vi "Read Configuration.vi"(0 "VISA resource name":refnum<visa-resource-name>, 11 "error in (no error)":errorcluster) -> (1 "function":i32(ring) items=["volts DC", "volts AC", "2-wire k.ohms", "4-wire k.ohms", "mA DC", "mA AC"], 3 "range":i32(ring) items=["200mV, 200 ohms", "2V, 2 kohms", "20V, 20 kohms", "200V, 200 kohms", "1000Vdc, 700 Vac, 2 Mohms", "20 Mohms"], 4 "VISA resource name out":refnum<visa-resource-name>, 6 "offset":bool, 10 "autorange":bool, 12 "rate":i32(ring) items=["slow", "medium", "fast"], 14 "trigger mode":i32(ring) items=["internal - continuous trigger", "external - rear panel trigger with delay", "external - bus trigger with delay", "external - rear panel trigger", "external - bus trigger"], 15 "error out":errorcluster)   [LabVIEW 2017, in "Fluke 8840.lvlib"]
doc: "This VI reads the current configuration of the multimeter."
uses:
  Fluke 8840.lvlib
panel:
  out "inputs":bool
  # "on\noff"
  # "rear\nfront"
  # "on\noff"
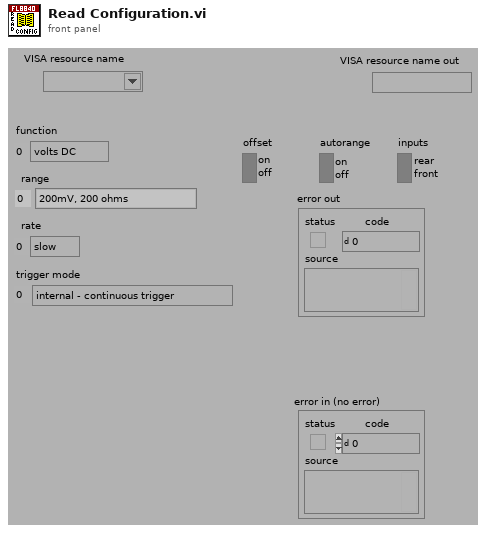
[diagram p1: front panel]
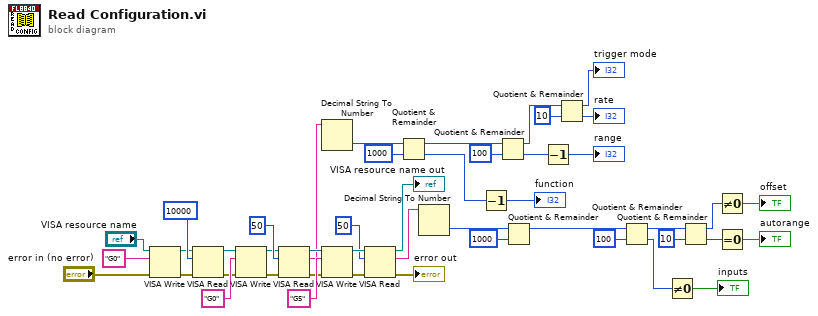
[diagram p0: block diagram]
diagram:
  n1 = VISA Write(VISA resource name="VISA resource name", write buffer="G0", error in (no error)="error in (no error)") -> (VISA resource name out=w4:refnum<visa-resource-name>, error out=w2:errorcluster)  [unwired: 1 out]
  n2 = VISA Read(VISA resource name=w4, byte count=u32 10000, error in (no error)=w2) -> (VISA resource name out=w3:refnum<visa-resource-name>, error out=w1:errorcluster)  [unwired: 2 out]
  n3 = VISA Write(VISA resource name=w3, write buffer="G0", error in (no error)=w1) -> (VISA resource name out=w13:refnum<visa-resource-name>, error out=w14:errorcluster)  [unwired: 1 out]
  n4 = VISA Read(VISA resource name=w13, byte count=u32 50, error in (no error)=w14) -> (VISA resource name out=w11:refnum<visa-resource-name>, read buffer=w10:string, error out=w12:errorcluster)  [unwired: 1 out]
  n5 = Decimal String To Number(string=w10) -> (number=w40:i32)  [unwired: 3 out]
  n6 = VISA Write(VISA resource name=w11, write buffer="G5", error in (no error)=w12) -> (VISA resource name out=w46:refnum<visa-resource-name>, error out=w45:errorcluster)  [unwired: 1 out]
  n7 = VISA Read(VISA resource name=w46, byte count=u32 50, error in (no error)=w45) -> (VISA resource name out=→"VISA resource name out":refnum<visa-resource-name>, read buffer=w9:string, error out=→"error out":errorcluster)  [unwired: 1 out]
  n8 = Quotient & Remainder(x=w40, y=1000) -> (x-y*floor(x/y)=w36:i32, floor(x/y)=w21:i32)
  n9 = Decimal String To Number(string=w9) -> (number=w27:i32)  [unwired: 3 out]
  n10 = Decrement(x=w21) -> (x-1=→"function":i32)
  n11 = Quotient & Remainder(x=w36, y=100) -> (x-y*floor(x/y)=w35:i32, floor(x/y)=w19:i32)
  n12 = Quotient & Remainder(x=w27, y=1000) -> (x-y*floor(x/y)=w29:i32)  [unwired: 1 out]
  n13 = Decrement(x=w19) -> (x-1=→"range":i32)
  n14 = Quotient & Remainder(x=w35, y=10) -> (x-y*floor(x/y)=→"trigger mode":i32, floor(x/y)=→"rate":i32)
  n15 = Quotient & Remainder(x=w29, y=100) -> (x-y*floor(x/y)=w28:i32, floor(x/y)=w26:i32)
  n16 = Not Equal To 0?(x=w26) -> (x != 0?=→"inputs":bool)
  n17 = Quotient & Remainder(x=w28, y=10) -> (x-y*floor(x/y)=w24:i32, floor(x/y)=w25:i32)
  n18 = Not Equal To 0?(x=w24) -> (x != 0?=→"offset":bool)
  n19 = Equal To 0?(x=w25) -> (x = 0?=→"autorange":bool)
